vi "NumberToString.vi"(8 "element 4":i32, 9 "element 3":i32, 10 "element 2":i32, 11 "element":i32) -> (0 "element 8":string, 1 "element 7":string, 2 "element 6":string, 3 "element 5":string)   [LabVIEW 2015]
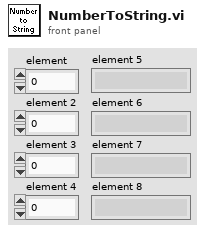
[diagram p1: front panel]
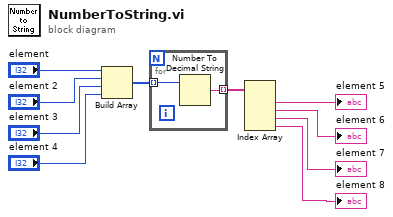
[diagram p0: block diagram]
diagram:
  n1 = Build Array("element", "element 2", "element 3", "element 4") -> (w6:i32[])
  n2 = for {
    tunnel: w6 -> [w12] mode=indexing
    tunnel: [w11] -> w5 mode=indexing
    n3 = Number To Decimal String(number=w12) -> (decimal integer string=w11:string)  [unwired: 1 in]
  }
  n4 = Index Array(array=w5) -> (element #1=→"element 5":string, element #2=→"element 6":string, element #3=→"element 7":string, element #4=→"element 8":string)  [unwired: 4 in]
